vi "20.vi"() -> ()   [LabVIEW 2020]
panel:
  out "Array":cluster{"Numeric":i32, "Array":bool[][]}[](array[cluster])
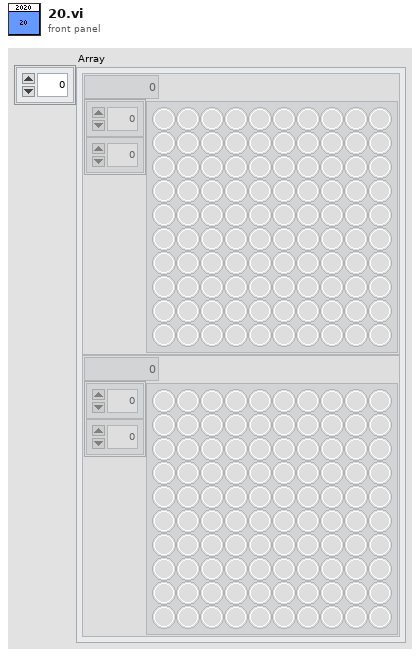
[diagram p1: front panel]
diagram:
  (unwired) "#" ("search string")
  (unwired) "#" ("search string")
  w7 = "Tile 3623:\n.##...#.#.\n..##..#...\n#......#.#\n#.#..#.#..\n##......#.\n......#..#\n###...#.#.\n#.#.#.#.#.\n......####\n#####....#\n\nTile 1301:\n.#..###..#\n.##..##..#\n#.......#.\n###...###.\n##.#..#.##\n.#.##.##..\n#.#####.##\n#..##.....\n#......#..\n...#...#..\n\nTile 3089:\n######.##.\n.#...#..##\n#.#.##.#.#\n#....#....\n#.....#..#\n#.##..#..#\n.##..#..#.\n#.##...##.\n#..#.###..\n#.###.#..#\n\nTile 3217:\n#.######..\n...#.#...#\n.#.#..#...\n#.#.##...#\n#..#..#...\n...#......\n..#..#.###\n#.#...##..\n#...#..#..\n..##.##..#\n\nTile 3203:\n.##...#..#\n#...##...#\n#....#....\n#.###....#\n#.##......\n.....#.#..\n....#....#\n#..#.....#\n#......#.#\n##.#.###..\n\nTile 3467:\n.#....#.#.\n...###...#\n#...#.####\n..###.#..#\n.....####.\n#...##.##.\n##.#.#.#..\n##....#..#\n##......#.\n#####..###\n\nTile 1013:\n#.....##..\n.#..#..###\n##....#.#.\n#.#.##.#.#\n###....#..\n#...#..#..\n#.##....#.\n...#......\n.......#..\n.##.#..#..\n\nTile 2843:\n.##.#...##\n#.###.#...\n#....##.#.\n#...###.#.\n.#..#.....\n.....##...\n###.##..#.\n...#..#...\n#.#....#..\n#.####..#.\n\nTile 1549:\n###...#...\n.#.##....#\n.......#..\n#.###...##\n##..#..#..\n.#.#......\n#.####...#\n#.##....##\n#.......#.\n#.#.###.#.\n\nTile 2591:\n######.#.#\n.###.....#\n#..####.##\n#..#..#..#\n...#.#.##.\n...###....\n.#...#..#.\n.##....#..\n...##....#\n##...#....\n\nTile 2897:\n###..##.#.\n...#..##..\n..........\n.....#...#\n....###..#\n...#.#...#\n#..###.#..\n.....#...#\n#....#....\n...#####..\n\nTile 3433:\n##...#....\n#.##.....#\n..##...##.\n#..##...#.\n#..#.#..##\n#.#....#..\n....##...#\n#..#......\n###.#.....\n.#.#.#..##\n\nTile 1153:\n#.#.##..##\n##..###...\n#..#.....#\n....#.#.##\n.#.#...#..\n#....#...#\n.#.....#..\n#..#..###.\n..#.#.##.#\n##...##...\n\nTile 1223:\n.#..###.#.\n.....#.#..\n....#....#\n..#.......\n##.###...#\n..#.#.#..#\n.##.......\n.##......#\n#........#\n......#...\n\nTile 1579:\n.##.####.#\n..........\n..........\n.........#\n##..#..#..\n#.##....#.\n##...#....\n#..#.#...#\n..##.#...#\n###..#..#.\n\nTile 2687:\n#..#.#....\n##...#....\n#...#.##..\n.....#..#.\n#.........\n#...#....#\n#....#...#\n..........\n##.....###\n###..#.###\n\nTile 3881:\n..##..###.\n##.#...#.#\n..#....#.#\n##........\n#........#\n#........#\n#..#...###\n#.##.#.#..\n.....#..##\n###...#.##\n\nTile 3169:\n...#.#####\n#.........\n.......##.\n.#..#.#...\n#.......#.\n...##....#\n#.#.#.#..#\n...#.#....\n#.......##\n.....##.##\n\nTile 1973:\n##..###...\n.#.#.##...\n#......#..\n#...#...##\n#..#.#..#.\n#.#.#..#.#\n.......##.\n.#.....#.#\n...#..###.\n##.#.#..#.\n\nTile 3581:\n####.###..\n..#......#\n..##.....#\n.#.####...\n...#..#.#.\n....#....#\n.#.....#..\n###.#.#...\n#......###\n##...#...#\n\nTile 1723:\n..####...#\n##........\n......#..#\n...#...#.#\n#.##.#..##\n#.....##.#\n..#......#\n..........\n...#.#...#\n#..#.##.#.\n\nTile 2539:\n#.##.#..##\n#....#...#\n#.##..#.##\n......##..\n.....#..##\n#....#...#\n......#..#\n###.###..#\n......#...\n..#.##..##\n\nTile 2531:\n....##.##.\n#..#.#..#.\n....#....#\n...##.#..#\n.##..#..#.\n.#....###.\n#.####.#.#\n....#..#.#\n###..##.##\n.#...##..#\n\nTile 3917:\n#.#...#...\n#.#.......\n.#.##.#...\n.##...#...\n..##.##.##\n#.....#...\n#...#...#.\n#.##.....#\n..#..#..#.\n#..##....#\n\nTile 1489:\n..#..#.###\n#...#####.\n....##...#\n.#.##.##.#\n.####....#\n...#...###\n..........\n#..##.#.#.\n##..#.#.#.\n#.##...###\n\nTile 1669:\n##.##.###.\n...#....##\n#.#.....##\n..#....#.#\n.#.#...#..\n####.##...\n#..###..#.\n#..##...##\n#.#.#.....\n######.#.#\n\nTile 2549:\n###.#.....\n......#.#.\n#.#...#..#\n#....##...\n...#...#.#\n##.......#\n##...#...#\n......#..#\n#.....#.##\n..#.#...#.\n\nTile 3797:\n.#####...#\n#..##.#..#\n##.###.#..\n##..##....\n..####....\n...#...#.#\n##..#.##.#\n....#....#\n.####.#...\n.....##.#.\n\nTile 2137:\n#.#..#.###\n..##....##\n....##...#\n##.#..#...\n.##.##.###\n##...#.#.#\n#.....#.#.\n..#..#...#\n##..#.###.\n#...##.##.\n\nTile 2087:\n#.#...##..\n..###.....\n##.#....#.\n#........#\n..#.#..#.#\n.#..#...##\n.##......#\n...#..#..#\n#.#..#....\n######..##\n\nTile 3929:\n...##.#.#.\n..#..#...#\n.#.###....\n.##.......\n...##.#.##\n#...###.#.\n#.##.#....\n#.#....##.\n.........#\n.###.#####\n\nTile 1907:\n#.###.#.#.\n#........#\n##.#.##..#\n...#...##.\n##.#....#.\n.....#..#.\n.###...##.\n.#.......#\n.#...###..\n#..#.#.##.\n\nTile 3923:\n..#..##...\n........#.\n#....###..\n.........#\n...#.###..\n#...####.#\n..##...#..\n.##......#\n#.....#...\n.#.....#.#\n\nTile 2833:\n###.#.##.#\n#..###...#\n##..#.....\n#..##.#...\n..#..#.#.#\n..##.....#\n#........#\n#...#.#...\n##..#...#.\n.#########\n\nTile 2143:\n#.##.##..#\n#..#.##..#\n..#....#.#\n##.#.#...#\n....#...#.\n#.........\n##...#.##.\n#.##.###.#\n....##...#\n#...##.#.#\n\nTile 2039:\n#.##..##..\n....##.#..\n#...#.##.#\n##.#.#....\n.......#..\n#.##....##\n.#..##.#..\n...##.....\n#...#....#\n##....#.#.\n\nTile 3943:\n#.#..#.#..\n##..#...##\n...#.#...#\n.###.#.##.\n..#...#.##\n....#..###\n#..#...#..\n#..#.##.##\n##.###...#\n##...#####\n\nTile 1697:\n.#..#####.\n#....####.\n.#.#.....#\n.........#\n..#......#\n.#.#.....#\n#..##.##..\n##.#....#.\n.##..#....\n#.##.#####\n\nTile 1621:\n..#.###..#\n...###..#.\n..........\n#........#\n##........\n#.##....#.\n#...#.....\n....#.#..#\n#.........\n.###.###..\n\nTile 2683:\n#..######.\n.#......#.\n....#.#..#\n##......#.\n...#.....#\n......#..#\n##.......#\n.#...#.###\n###.#....#\n##.###.#.#\n\nTile 2203:\n##..##...#\n..#..#...#\n##...#....\n##..##....\n#...###..#\n...#..#.##\n#.....##.#\n..#...#..#\n###....#..\n####.#..#.\n\nTile 3469:\n###...##.#\n#.#..#####\n..#.#.#..#\n#..#......\n#...#....#\n##....#..#\n#...##....\n.#.#.###..\n..#..##.#.\n..##.#.#.#\n\nTile 1801:\n..#....#.#\n#...#..#..\n.#..#....#\n##..#.#.#.\n##.###.#.#\n..##..#...\n##..##....\n..#...####\n#.#.....#.\n.#.......#\n\nTile 3373:\n#.#..#..#.\n....##.#..\n#......###\n#....###.#\n##.#.#####\n#..#...##.\n#.##....#.\n.##.....#.\n......#...\n##..##.##.\n\nTile 2237:\n.###.#....\n..#..##..#\n#.#.##.#..\n#.#.##..#.\n...#..#..#\n#.##...#..\n####...###\n#..#.....#\n..#.....##\n###..#..##\n\nTile 2221:\n#.###.....\n...##.....\n..#.#.....\n#..##.....\n......#.##\n.....#.#..\n.#.#.....#\n....###...\n#....#.##.\n##.#####.#\n\nTile 2927:\n#.###...##\n......##..\n.......###\n##....##.#\n..#...#...\n..#...#.##\n#..#...#..\n.........#\n.#..#...##\n.####.#.#.\n\nTile 1861:\n.#.#...#..\n..#.......\n##.....#..\n#....#....\n##..#....#\n.##.#.##.#\n....##..##\n##.#....#.\n#.....###.\n#..#.....#\n\nTile 1097:\n#......#.#\n#....##..#\n###.#..###\n...#......\n..#....#.#\n#...#.....\n##..##.#.#\n###...##..\n#..##...##\n..###....#\n\nTile 3331:\n#..##.#..#\n#.###.##.#\n.#.##...#.\n...#.##..#\n.........#\n......##..\n#..#.....#\n..#....###\n...#.....#\n.##.#.##.#\n\nTile 1033:\n#.##..#.##\n..#.......\n...#...#..\n....##.###\n##.####..#\n#.#.##.##.\n.#..#..#..\n.........#\n#.#.......\n##.####..#\n\nTile 1933:\n..##....##\n#...#.##.#\n##....####\n......#.#.\n......###.\n#...#..###\n#...#.....\n......##..\n......#..#\n#....###..\n\nTile 1483:\n#.###....#\n#.###...##\n..........\n..#.#.#..#\n........##\n....#.....\n#.##.#...#\n....##....\n....#.##..\n....#..#..\n\nTile 3823:\n#.###.###.\n.##..#.##.\n#...#..#..\n#.##....#.\n....#.....\n###.####.#\n.#.##.#.##\n...##..#..\n#..#.#..#.\n..#.##..#.\n\nTile 1759:\n#..##...#.\n.####..###\n#.#......#\n.##...#..#\n##........\n##......##\n#..##....#\n..#...##..\n#......#.#\n####.#..##\n\nTile 1187:\n.##.#..###\n....##....\n##.#......\n#..##....#\n#.#.#.#.#.\n..#.###...\n....##...#\n..##.#..##\n#.#...#...\n..#.##..##\n\nTile 2857:\n..#.....#.\n..#..##..#\n##.#..#..#\n..#..###.#\n#........#\n...##....#\n#...#...#.\n##.....#.#\n##...##...\n#.#..#....\n\nTile 1811:\n.#.######.\n#.......#.\n....#..###\n##.....#..\n###....#..\n..#.#..##.\n#....#..##\n#......##.\n#.#....##.\n...#...###\n\nTile 1511:\n##.#.#####\n.....#..##\n#....#.#.#\n..#..##..#\n#.......#.\n#..##....#\n###.#.##.#\n#.......##\n###...#.#.\n.##....#..\n\nTile 2999:\n#####.####\n##.......#\n..#...#.#.\n.....#.##.\n.....#..#.\n.......###\n#.....#...\n#....#....\n#...####..\n###.#...##\n\nTile 3209:\n..#####...\n#.#.#....#\n#...#...##\n##........\n.....##.#.\n#..##.....\n..#.#.##.#\n##..##...#\n#.#......#\n#..#.#.#..\n\nTile 2273:\n#####..#.#\n...###...#\n#..##....#\n#......#.#\n..##.....#\n##.....#.#\n#..#..#.##\n#...##....\n........#.\n##.#.####.\n\nTile 1583:\n#.###.##..\n.#.#.#.#..\n........##\n...##...#.\n##..#.#..#\n...#.....#\n#........#\n.....##...\n######.###\n#.#..#.#.#\n\nTile 1787:\n###.#####.\n#...#.#..#\n#........#\n.#..##....\n...#..#..#\n#.#...#...\n#....#....\n.#....#..#\n#.#.#....#\n####.#.#.#\n\nTile 3323:\n###..##...\n#.....##..\n#...###...\n##..##..##\n#..#.#.#.#\n.......##.\n#...#....#\n.....#.#..\n..#.#..#..\n#.##.###..\n\nTile 1429:\n...##..#.#\n..........\n....#..#.#\n.........#\n.#.......#\n.##....#..\n...#.#..#.\n.#.#..#..#\n####.##...\n#.#######.\n\nTile 3221:\n...#..#..#\n#..#..##..\n....###.#.\n######...#\n....#..#..\n#....#.#..\n###..#...#\n.........#\n#....##..#\n###.#.###.\n\nTile 3299:\n###.###..#\n...#.#.##.\n#...##....\n.....#..#.\n...#.....#\n#.#.......\n#....#..#.\n.#.#.....#\n...#.....#\n.##...####\n\nTile 1741:\n#..##.##.#\n.##..#..##\n#.###..##.\n#.......#.\n##.....#.#\n#..#.#....\n##.#..##..\n####.##.##\n#........#\n.###.#...#\n\nTile 1063:\n##.##...#.\n.#..##....\n...#...#..\n#.#.....##\n.##....#..\n#.#.#.....\n####.#..##\n.#.##.....\n.#.##....#\n#.#..##.#.\n\nTile 2381:\n...####.##\n#.#.##...#\n....#.....\n.#..#.##.#\n##.###.#..\n###......#\n#.....#...\n##.####...\n..#...####\n#.####.##.\n\nTile 3463:\n.###.#.#..\n####.#.###\n.#..#.....\n##........\n#.##...#.#\n.#........\n#...#...#.\n......#..#\n##.#..#...\n..#..#..##\n\nTile 2063:\n#..#.#.###\n#.##.....#\n..#....#..\n.#...#..##\n.####...##\n##..##.#..\n.........#\n..##......\n#....#...#\n...##...#.\n\nTile 1487:\n##..##.###\n#........#\n....#....#\n.....#..##\n#....#....\n#.#...#.#.\n#....#.#..\n.#..##...#\n.#...#.#.#\n#..####.#.\n\nTile 2243:\n.#..#.#.#.\n###...#...\n...##.....\n.#...###..\n.#.#..##..\n#..###..##\n..#..##.##\n..##.....#\n....#.#...\n.....#####\n\nTile 1657:\n##...#.#..\n#...####..\n#...##.#..\n......#.##\n..#.....##\n###....###\n##.#.##...\n.#.#...#..\n#........#\n..####.###\n\nTile 2081:\n########..\n#.#.#...##\n#.#...#...\n###.#.#.#.\n#.......#.\n...#.#....\n##........\n#.##.#..#.\n#.###.....\n..#.#.###.\n\nTile 2287:\n######..##\n#......#..\n....#.....\n#..#.#....\n##...#....\n#..#....##\n#....#....\n#.........\n#..#....#.\n......###.\n\nTile 1181:\n.####.##.#\n..#....###\n#.........\n.....#....\n.##..#.##.\n#####..#..\n...#..###.\n##...#.#..\n#..#.##...\n..#.#....#\n\nTile 3041:\n##..#.####\n#..#....#.\n#.#..#..#.\n#....#...#\n#........#\n#.....#...\n##..#.....\n..####..#.\n..##....##\n.#.####.##\n\nTile 1319:\n###.#...##\n##....#...\n.....##.##\n...#.###.#\n#......#..\n##..#.....\n##...##.#.\n...#...#..\n#.###.#.#.\n.######...\n\nTile 3271:\n...##.####\n#.......#.\n.#........\n#......#.#\n..#..#..##\n#.##.....#\n...#..#.#.\n.####..###\n.....##..#\n.#.##..##.\n\nTile 1279:\n#..#.#.#..\n#.##..#..#\n##....#..#\n..#.#....#\n#.#...#...\n.##....#..\n###.#....#\n....#...#.\n.#....#.#.\n########..\n\nTile 2029:\n.#.....#.#\n##.#.....#\n..##....#.\n.#.###.#..\n.#....#.#.\n#........#\n.......###\n#......##.\n..#.#.#...\n#..#..#.##\n\nTile 3361:\n###.#.#.#.\n...#...#..\n#.#.#....#\n#.......#.\n....#..##.\n#.##....##\n..##..#.##\n#..#...#.#\n..#...#..#\n..##.##..#\n\nTile 3889:\n####.##.#.\n#..#....#.\n...##....#\n#...#...#.\n..#......#\n..####...#\n#.#..####.\n##.......#\n...#...#.#\n#.#...##.#\n\nTile 2459:\n...#.#.#.#\n..#......#\n...##.#...\n.#..##...#\n.#...#..##\n.#....#..#\n##.......#\n##.#......\n#.#.#.##.#\n##..#.###.\n\nTile 1951:\n.#.###.###\n...#.#.###\n#.......#.\n..##.....#\n...#...#..\n#.#..##...\n#.##......\n#..#.###..\n...###...#\n#.....####\n\nTile 1627:\n#.##......\n#.#..#.#..\n.##.......\n.###....##\n##..#..#..\n..#....#.#\n.##..#....\n##.#.#....\n##.......#\n.##.#.#..#\n\nTile 1297:\n##.#...#..\n#....#.#.#\n.......#..\n##......#.\n#...#.....\n#........#\n.....#.#.#\n.#....#.#.\n#..#..#..#\n########.#\n\nTile 3989:\n...#......\n....#...#.\n###.......\n.#...###.#\n##.#......\n.#..#....#\n.#...#.#.#\n..#####..#\n##....##.#\n.#.#...###\n\nTile 3779:\n#.#.##.#..\n#.#......#\n...#.....#\n.#...#.#..\n...##.#...\n#..#..##.#\n#....##...\n###.#....#\n.##..##..#\n...##....#\n\nTile 3769:\n....#..#..\n##.#....#.\n.#.##..#.#\n#.##.#..##\n....#.##..\n#.....##..\n#....##.#.\n#.#.###.#.\n##.#.###.#\n.#...##...\n\nTile 3803:\n#..#######\n.#..###...\n..#..#.###\n##..#.#...\n.###.....#\n##........\n#######...\n#.#.##....\n....#....#\n##....#.#.\n\nTile 1777:\n..#.##.##.\n#.....#..#\n....#..##.\n..#..#...#\n#....###.#\n#....#..#.\n.........#\n#.....#..#\n#.....#.#.\n##.###..##\n\nTile 1663:\n#.##..###.\n#..#.#...#\n.....#...#\n..##.##...\n#..##.....\n#...#..#.#\n#...#.#...\n##.#.#...#\n#.####...#\n......#..#\n\nTile 3329:\n..##.#...#\n.#........\n..##..##..\n#...##.###\n#.#.#..#.#\n#..#.#...#\n.....#.###\n.##..#.#.#\n.###..##..\n#####....#\n\nTile 1459:\n.#.....###\n..........\n#....#....\n........#.\n...##..###\n...#......\n.#..#.##.#\n..#..#.###\n#.#......#\n.#.#...###\n\nTile 3343:\n.##.##....\n.##.#.####\n#..#..#.#.\n#.###....#\n..#..#....\n#.......##\n#.#....##.\n#........#\n...#...#.#\n...##...##\n\nTile 3793:\n##.##....#\n..##.....#\n#..#..##.#\n#...###.##\n##........\n#......#.#\n.##....#..\n#.#.#.....\n...#....#.\n#...##.###\n\nTile 3527:\n###.#....#\n#.#.##.#..\n.#...#....\n.........#\n#......#.#\n#.......##\n...#.#....\n....#...#.\n#.....#.##\n.#.######.\n\nTile 1721:\n.###.#..##\n#.###....#\n#.#.#....#\n##.#....#.\n#.#...#..#\n.#..#####.\n##.#......\n..#.###.#.\n#......#.#\n#.##....#.\n\nTile 2357:\n##.##.#..#\n..#.....#.\n...#.#....\n##.......#\n#.#.#..#.#\n#.#...#.##\n##.....#..\n#.....#...\n#..##.....\n#..######.\n\nTile 2207:\n.##...###.\n##..#.#.##\n##..###..#\n..#.###.##\n...###...#\n#..#.....#\n.#.###....\n.#..#.#...\n#####...#.\n.#...#...#\n\nTile 2633:\n##.#.....#\n.....#..##\n......#.##\n#........#\n...###....\n..#.#..#.#\n#....#...#\n##...#..#.\n.#..#..###\n######.##.\n\nTile 3253:\n##...#.#..\n.##.###.#.\n#.......#.\n....###..#\n##.#..#...\n...#.....#\n#.....##.#\n....#.....\n##..##.#..\n##..##.#.#\n\nTile 2293:\n#.#..#...#\n#.......##\n#.#.#....#\n#...##.##.\n#.##.#....\n#..#.#....\n#.#.......\n#........#\n#........#\n.#.#......\n\nTile 2671:\n##.#.#...#\n..##...#..\n####...#..\n##....#...\n#...#....#\n.....#..#.\n.#.#..#.##\n###.####.#\n#.####.#.#\n###.###.#.\n\nTile 3119:\n........#.\n...##...#.\n#.#....##.\n.#...#....\n...#...##.\n.###..#..#\n.........#\n#.#....#..\n.#.......#\n##......#.\n\nTile 3413:\n.......#.#\n##...#...#\n......###.\n#.#.......\n##.#.....#\n#..#....##\n##..#...#.\n..#.#.####\n.#.....#.#\n.....####.\n\nTile 2969:\n...######.\n.#.#....#.\n#.#....#.#\n....###.##\n.....#.#..\n..###..#.#\n#.##....#.\n..###.#...\n..#.......\n.......#.#\n\nTile 2713:\n..#.#.#...\n...#......\n.....#....\n.###.#...#\n#..#......\n#.#.###..#\n#...##..##\n###....##.\n...#.##.#.\n##..#..#.#\n\nTile 2749:\n#.....#..#\n.##.#...##\n#..#....#.\n..##..#...\n.#..##...#\n###..#...#\n..#....#.#\n#...##.###\n#..#.....#\n#.##..#...\n\nTile 1117:\n...#..##.#\n.....##...\n...#.#..##\n#.#.#....#\n#.#...#...\n.#######..\n.#.#..###.\n#...#.##.#\n##....#...\n..####..##\n\nTile 3517:\n########.#\n###..#.###\n#.........\n.#.....###\n##...#...#\n.#..#..#..\n.##.####.#\n......#..#\n.....##..#\n...#...#.#\n\nTile 1523:\n#..####.#.\n.#.....#..\n#.#.......\n....#.....\n.....####.\n#.#....##.\n.#.....##.\n.#..#.....\n..#...#..#\n###...####\n\nTile 2879:\n.##...#...\n##....####\n..###...#.\n.###.##..#\n....##....\n...##.....\n##.#.#.#.#\n#.#....##.\n#..#......\n###..#####\n\nTile 3851:\n##.#.#.#.#\n......##..\n#....##.#.\n##...#....\n#..#..#.#.\n....#####.\n###.##...#\n#...###.#.\n#........#\n.#..#..##.\n\nTile 2659:\n##...####.\n.........#\n.###..#.##\n#...###.#.\n#.##.....#\n#####...##\n..#......#\n##.#......\n##...##...\n#.....####\n\nTile 1171:\n#.....#.##\n.#...#....\n.#...#...#\n#...#...#.\n#....#...#\n....#...#.\n.#..#.#.##\n#....#.#.#\n.#...#...#\n##.......#\n\nTile 2711:\n....#.###.\n#....#.###\n#..#..#.##\n......#.#.\n.#.#......\n#.#....#.#\n#.......##\n...#......\n.....#.#.#\n......#..#\n\nTile 1543:\n#..#..###.\n..#.......\n...#.#.#.#\n#..#....#.\n#.#.#....#\n.##....###\n..#..#...#\n..#.#...#.\n...#..#...\n#####..##.\n\nTile 3163:\n#.#.#.##..\n........#.\n..##.###..\n#..#...#..\n..#.#..#..\n#.....###.\n.#........\n......#.#.\n..#.#..#..\n#.##.#...#\n\nTile 1249:\n#....###.#\n..#.###...\n##...#..##\n.#..#...#.\n#.#.......\n#......#.#\n#.......##\n..........\n#........#\n.##.###.#.\n\nTile 2003:\n#.#..#..##\n#..#.....#\n#...#.##..\n...###.##.\n..#.#.....\n#.##...#..\n........##\n###.#.#..#\n.#.....#..\n#.##.#.#..\n\nTile 2129:\n#.....##..\n.#...#...#\n...#.....#\n.....#.#.#\n...##.#...\n#.........\n...#.#...#\n.....##.##\n...#..#..#\n.####.#..#\n\nTile 3391:\n.#.#...#..\n#..#..#...\n......#..#\n#..#.#.#..\n.#...##..#\n#.#..#...#\n....#....#\n#.....#.##\n#........#\n..##..####\n\nTile 1867:\n.##..##.##\n....#...#.\n##.#..#...\n..##......\n###.....#.\n#........#\n##.#...#.#\n.#.#..##..\n#.#...#...\n##......#.\n\nTile 1747:\n###..##.##\n#...#.#.#.\n..##......\n#..####...\n.#.###.##.\n#......#.#\n#...#.....\n...##....#\n.#.#......\n#.#...##..\n\nTile 3191:\n#...#...#.\n..###.....\n#.##.#....\n.##...#...\n#.###.##..\n##.##..###\n.###..####\n#....#..#.\n.....#....\n.##.####..\n\nTile 3511:\n.##.##.###\n#.#.#.##.#\n....#...##\n....#...#.\n#.##.#.#..\n##...##..#\n#.#....#.#\n#.#...#...\n..........\n....#.#.#.\n\nTile 2657:\n####..##.#\n.#..#...##\n....#.##.#\n.......#..\n#.#..#....\n.#.#..#.##\n######....\n.....##..#\n...#..##.#\n#.#.####.#\n\nTile 3697:\n#####.#..#\n#.##.#..#.\n##.##..#..\n#.#.##..#.\n##.####..#\n.###.....#\n.#....##.#\n..#.##..#.\n#.........\n##..###.#.\n\nTile 1123:\n.....#...#\n#.......##\n##.#..##.#\n..........\n..##......\n...#..##.#\n####.....#\n.##......#\n##........\n.#.......#\n\nTile 2729:\n.##....###\n#...###.#.\n###.#...##\n#.##...#..\n##......##\n....#...##\n#.....#...\n#.##..###.\n....#.#...\n#..####.##\n\nTile 3533:\n..#.##..#.\n..##.#...#\n#....##..#\n#.....##..\n#.....#..#\n..........\n#..#..##..\n#.....##..\n.#..##...#\n.##.#.#.#.\n\nTile 3919:\n#...#.....\n#....###..\n.....###..\n##...#...#\n.#..##....\n..##...#.#\n.........#\n..#.###...\n##........\n####.##...\n\nTile 1453:\n#.....##.#\n#.......#.\n.#.#..#.##\n#....#...#\n......##..\n....#....#\n..#..#..##\n##..#.##.#\n#....##...\n#####.##.#\n\nTile 3643:\n..#.#.####\n.........#\n#...#.##.#\n...##...##\n.#......##\n#.#....#..\n.#........\n#.#.#....#\n####.....#\n###.####..\n\nTile 2767:\n.##..####.\n...#...#..\n..#......#\n....#.####\n.#.#..#.#.\n#.....#.#.\n##..#...#.\n#.###.#...\n#...##...#\n...##.#.#.\n\nTile 3541:\n##.##...##\n#.....##.#\n#........#\n.#..##....\n#......#..\n......#..#\n#....#..#.\n.#.#.#.#..\n###..#..#.\n#.######..\n\nTile 3617:\n###..#....\n#..#......\n.......##.\n....#...##\n#...#..#..\n.#..#...#.\n#..#.#..#.\n.........#\n#...#..#.#\n#..#.#..#.\n\nTile 1229:\n.#...#.##.\n.......#..\n#.#.#.#.##\n###..#...#\n#.#..#...#\n...##.#..#\n.#.#......\n#....#...#\n#..#..####\n#.##..###.\n\nTile 1259:\n#..##.####\n.........#\n.#...####.\n#.#..#...#\n#.#...#.##\n#...#.#.#.\n......#..#\n#.........\n....#.....\n.##..####."
  n1 = call <userlib>:"Multi-line String to Array__ogtk.vi"("string"=w7) -> ("lines"=w3:string[])
  n2 = Search and Replace String(replace all?=TRUE ("replace all? (F)"), input string=w7, search string="Tile") -> (number of replacements=w4:i32)  [unwired: 5 in, 3 out]
  n3 = for {
    N: w4 -> [_]
    tunnel: w3 -> [w20]
    tunnel: 35 ("length") -> [w11]
    tunnel: [w9] -> w1 mode=indexing
    i -> [w19]
    n4 = expression code="x*12"(w19) -> (w18:i32)
    n5 = Array Subset(array=w20, index=w18, length=11) -> (w16:string[])
    n6 = Delete From Array(array=w16, index=0) -> (deleted portion=w14:string, array with subset deleted=w12:string[])  [unwired: 1 in]
    n7 = for {
      tunnel: w12 -> [w24] mode=indexing
      tunnel: w11 -> [w22]
      tunnel: [w21] -> w10 mode=indexing
      n8 = String To Byte Array(string=w24) -> (unsigned byte array=w23:u8[])
      n9 = Equal?(x=w23, y=w22) -> (x = y?=w21:bool[])
    }
    n10 = Scan From String(format string="Tile %d:", input string=w14) -> (output 1=w8:i32)  [unwired: 3 in, 3 out]
    n11 = case shown="0, Default" w8 {
      frame 0, Default {
      }
      frame 1.. {
      }
    }
    n12 = Bundle(w8, w10) -> (w9:cluster{i32, bool[][]})  [unwired: 1 in]
  }
  "Array" <- w1
